vi "Server_API_Call.vi"(6 "Server":path, 7 "Direction":enum16{"ASK", "TELL"}(ring), 8 "error in (no error)":errorcluster, 9 "Payload":string, 11 "cmd":string) -> (0 "error out":errorcluster, 1 "Running?":bool, 3 "Read from Server":string)   [LabVIEW 2020]
panel:
  in  "port":refnum<visa-resource-name>
  out "Script Running?":bool
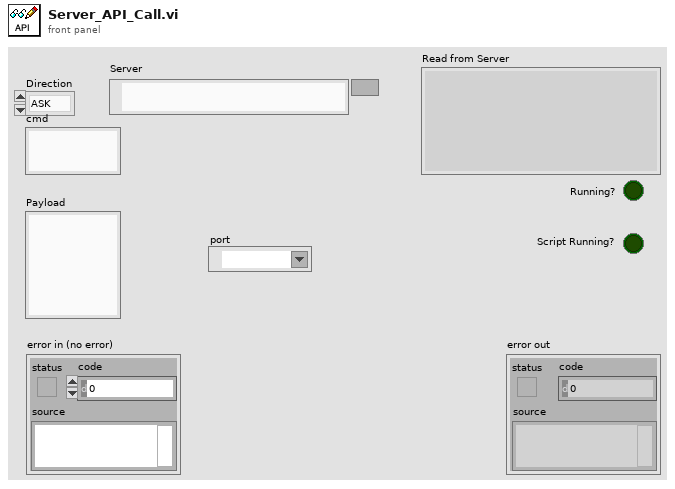
[diagram p1: front panel]
types:
  T1 = enum32{"Bad", "Idle", "Run top level", "Running"}
  T2 = enum32{"Invalid", "Standard", "Closed", "Hidden", "Minimized", "Maximized"}
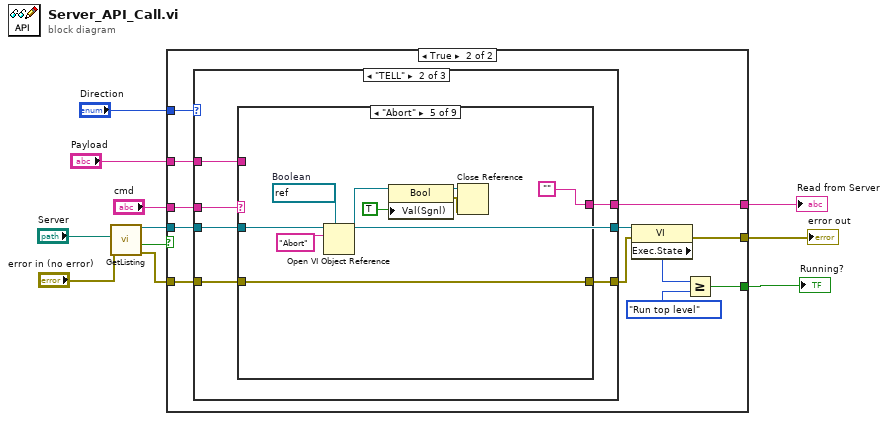
[diagram p0: block diagram]
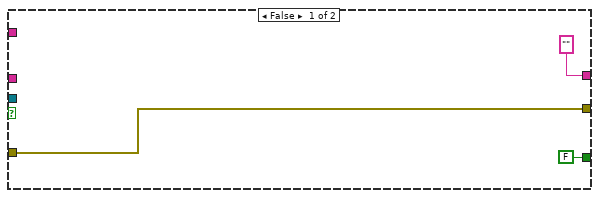
[diagram p2: hidden frame]
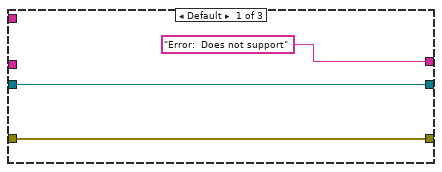
[diagram p3: hidden frame]
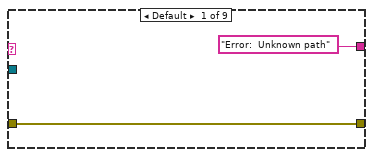
[diagram p4: hidden frame]
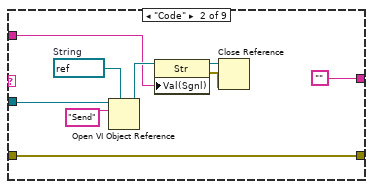
[diagram p5: hidden frame]
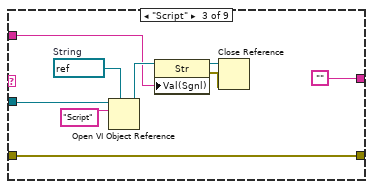
[diagram p6: hidden frame]
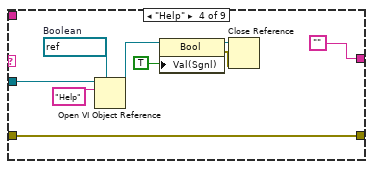
[diagram p7: hidden frame]
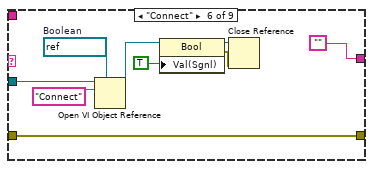
[diagram p8: hidden frame]
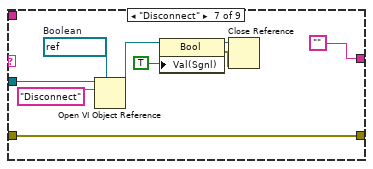
[diagram p9: hidden frame]
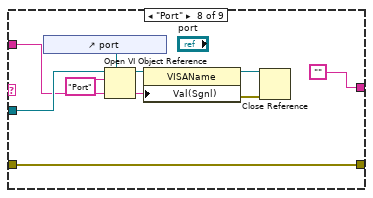
[diagram p10: hidden frame]
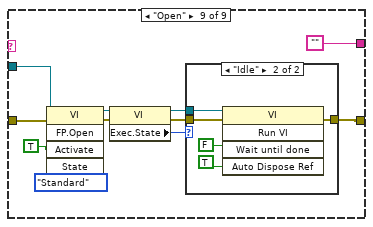
[diagram p11: hidden frame]
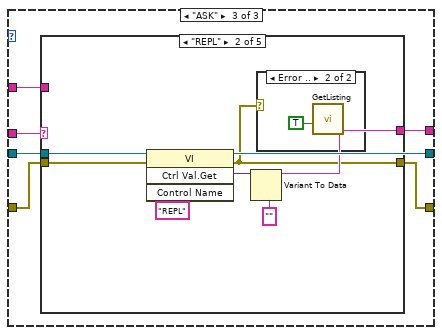
[diagram p13: hidden frame]
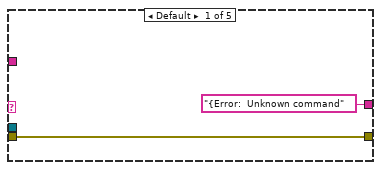
[diagram p14: hidden frame]
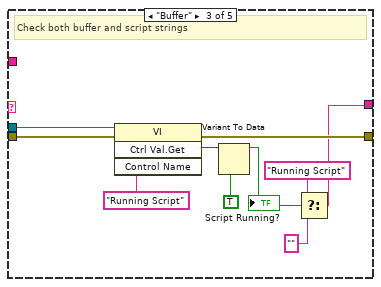
[diagram p16: hidden frame]
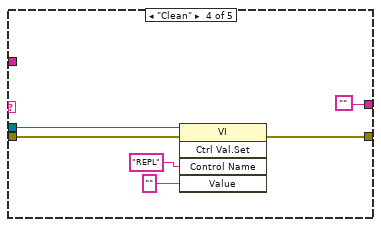
[diagram p17: hidden frame]
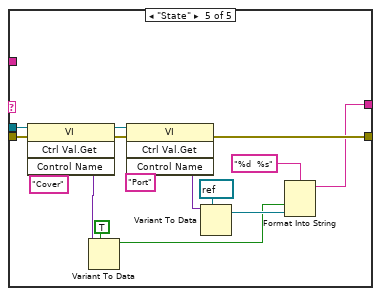
[diagram p18: hidden frame]
diagram:
  n1 = call "GetListing.vi"("error in (no error)"="error in (no error)", "Server"="Server") -> ("error out"=w4:errorcluster, "Found"=w1:bool, "VI out"=w9:refnum<vi>)  [unwired: 7 in]
  n2 = case shown="True" w1 {
    tunnel: ["" ("input 2") w26] -> w11
    tunnel: w9 -> [_ w25]
    tunnel: "Direction" -> [_ w24]
    tunnel: "Payload" -> [_ w23]
    tunnel: "cmd" -> [_ w22]
    tunnel: w4 -> [w13 w21]
    tunnel: [FALSE w16] -> w3
    tunnel: [w13 w15] -> w2
    frame False {
    }
    frame True {
      n3 = case shown="\"TELL\"" w24 {
        tunnel: ["Error:  Does not support" ("input 2") w35 w123] -> w26
        tunnel: w23 -> [_ w34 w122]
        tunnel: w25 -> [w27 w30 w118]
        tunnel: w21 -> [w28 w33 w121]
        tunnel: [w28 w32 w120] -> w19
        tunnel: w22 -> [_ w31 w119]
        tunnel: [w27 w30 w118] -> w20
        frame Default {
        }
        frame "TELL" {
          n4 = case shown="\"Abort\"" w31 {
            tunnel: ["Error:  Unknown path" ("input 2") "" "" "" "" "" "" "" ""] -> w35
            tunnel: w34 -> [_ w40 w49 _ _ _ _ w92 _]
            tunnel: w33 -> [w36 w45 w54 w64 w73 w82 w91 w100 w107]
            tunnel: [w36 w45 w54 w64 w73 w82 w91 w100 w101] -> w32
            tunnel: w30 -> [_ w42 w51 w61 w70 w79 w88 w98 w108]
            frame Default {
            }
            frame "Code" {
              w44 = refnum<vi> refnum  # String
              n5 = Open VI Object Reference(7:w44, 10:"Send" ("name/order"), 11:w42) -> (3:w41:refnum<vi>)  [unwired: 1 in, 1 out]
              n6 = property class="Str"(reference=w41, "Val(Sgnl)"=w40) -> (reference out=w38:refnum<vi>, error out=w39:errorcluster)  [unwired: 1 in]
              n7 = Close Reference(reference=w38, error in (no error)=w39) -> ()  [unwired: 1 out]
            }
            frame "Script" {
              w53 = refnum<vi> refnum  # String
              n8 = Open VI Object Reference(7:w53, 10:"Script" ("name/order"), 11:w51) -> (3:w50:refnum<vi>)  [unwired: 1 in, 1 out]
              n9 = property class="Str"(reference=w50, "Val(Sgnl)"=w49) -> (reference out=w47:refnum<vi>, error out=w48:errorcluster)  [unwired: 1 in]
              n10 = Close Reference(reference=w47, error in (no error)=w48) -> ()  [unwired: 1 out]
            }
            frame "Help" {
              w63 = refnum<vi> refnum  # Boolean
              n11 = Open VI Object Reference(7:w63, 10:"Help" ("name/order"), 11:w61) -> (3:w60:refnum<vi>)  [unwired: 1 in, 1 out]
              n12 = property class="Bool"(reference=w60, "Val(Sgnl)"=TRUE) -> (reference out=w58:refnum<vi>, error out=w59:errorcluster)  [unwired: 1 in]
              n13 = Close Reference(reference=w58, error in (no error)=w59) -> ()  [unwired: 1 out]
            }
            frame "Abort" {
              w72 = refnum<vi> refnum  # Boolean
              n14 = Open VI Object Reference(7:w72, 10:"Abort" ("name/order"), 11:w70) -> (3:w69:refnum<vi>)  [unwired: 1 in, 1 out]
              n15 = property class="Bool"(reference=w69, "Val(Sgnl)"=TRUE) -> (reference out=w67:refnum<vi>, error out=w68:errorcluster)  [unwired: 1 in]
              n16 = Close Reference(reference=w67, error in (no error)=w68) -> ()  [unwired: 1 out]
            }
            frame "Connect" {
              w81 = refnum<vi> refnum  # Boolean
              n17 = Open VI Object Reference(7:w81, 10:"Connect" ("name/order"), 11:w79) -> (3:w78:refnum<vi>)  [unwired: 1 in, 1 out]
              n18 = property class="Bool"(reference=w78, "Val(Sgnl)"=TRUE) -> (reference out=w76:refnum<vi>, error out=w77:errorcluster)  [unwired: 1 in]
              n19 = Close Reference(reference=w76, error in (no error)=w77) -> ()  [unwired: 1 out]
            }
            frame "Disconnect" {
              w90 = refnum<vi> refnum  # Boolean
              n20 = Open VI Object Reference(7:w90, 10:"Disconnect" ("name/order"), 11:w88) -> (3:w87:refnum<vi>)  [unwired: 1 in, 1 out]
              n21 = property class="Bool"(reference=w87, "Val(Sgnl)"=TRUE) -> (reference out=w85:refnum<vi>, error out=w86:errorcluster)  [unwired: 1 in]
              n22 = Close Reference(reference=w85, error in (no error)=w86) -> ()  [unwired: 1 out]
            }
            frame "Port" {
              n23 = control-ref of="port"() -> (w93:refnum<vi>)
              n24 = Open VI Object Reference(7:w93, 10:"Port" ("name/order"), 11:w98) -> (3:w97:refnum<vi>)  [unwired: 1 in, 1 out]
              n25 = property class="VISAName"(reference=w97, "Val(Sgnl)"=w92) -> (reference out=w95:refnum<vi>, error out=w96:errorcluster)  [unwired: 1 in]
              n26 = Close Reference(reference=w95, error in (no error)=w96) -> ()  [unwired: 1 out]
            }
            frame "Open" {
              n27 = invoke class="VI" method="FP.Open"(reference=w108, error in=w107, "Activate"=TRUE ("Activate?"), "State"=T2."Standard" ("Front Panel Window:State")) -> (reference out=w106:refnum<vi>, error out=w105:errorcluster)  [unwired: 1 in, 3 out]
              n28 = property class="VI"(reference=w106, error in=w105) -> (reference out=w103:refnum<vi>, error out=w102:errorcluster, "Exec.State"=w104:T1)
              n29 = case shown="\"Idle\"" w104 {
                tunnel: w103 -> [_ w117]
                tunnel: w102 -> [w112 w116]
                tunnel: [w112 w115] -> w101
                frame Default {
                }
                frame "Idle" {
                  n30 = invoke class="VI" method="Run VI"(reference=w117, error in=w116, "Wait until done"=FALSE ("Activate?"), "Auto Dispose Ref"=TRUE ("Activate?")) -> (error out=w115:errorcluster)  [unwired: 1 in, 4 out]
                }
              }
            }
          }
        }
        frame "ASK" {
          n31 = case shown="\"REPL\"" w119 {
            tunnel: ["{Error:  Unknown command" ("input 2") w127 w135 "" w150] -> w123
            tunnel: w122 -> [_ _ _ _ _]
            tunnel: w118 -> [_ w128 w140 w146 w158]
            tunnel: w121 -> [w124 w129 w134 w145 w157]
            tunnel: [w124 w126 w141 w144 w154] -> w120
            frame Default {
            }
            frame "REPL" {
              n32 = invoke class="VI" method="Ctrl Val.Get"(reference=w128, error in=w129, "Control Name"="REPL") -> (error out=w126:errorcluster, "Get Control Value Variant"=w131:variant)  [unwired: 1 in, 2 out]
              n33 = Variant To Data(type="" ("Control Name"), Variant=w131) -> (data=w127:string)  [unwired: 1 in, 1 out]
              n34 = case shown="Error .." w126 {
                frame No Error {
                }
                frame Error {
                  n35 = call "GetListing.vi"("Reset?"=TRUE) -> ()  [unwired: 8 in, 3 out]
                }
              }
            }
            frame "Buffer" {
              # "Check both buffer and script strings"
              n36 = invoke class="VI" method="Ctrl Val.Get"(reference=w140, error in=w134, "Control Name"="Running Script") -> (error out=w141:errorcluster, "Get Control Value Variant"=w142:variant)  [unwired: 1 in, 2 out]
              n37 = Variant To Data(type=TRUE, Variant=w142) -> (data=w138:bool)  [unwired: 1 in, 1 out]
              "Script Running?" <- w138
              n38 = Select(t="Running Script" ("Control Name"), s=w138, f="" ("Control Name")) -> (s? t:f=w135:string)
            }
            frame "Clean" {
              n39 = invoke class="VI" method="Ctrl Val.Set"(reference=w146, error in=w145, "Control Name"="REPL", "Value"="" ("Control Name")) -> (error out=w144:errorcluster)  [unwired: 1 in, 4 out]
            }
            frame "State" {
              n40 = invoke class="VI" method="Ctrl Val.Get"(reference=w158, error in=w157, "Control Name"="Cover") -> (reference out=w156:refnum<vi>, error out=w155:errorcluster, "Get Control Value Variant"=w159:variant)  [unwired: 1 in, 1 out]
              n41 = Variant To Data(type=TRUE, Variant=w159) -> (data=w151:bool)  [unwired: 1 in, 1 out]
              n42 = invoke class="VI" method="Ctrl Val.Get"(reference=w156, error in=w155, "Control Name"="Port") -> (error out=w154:errorcluster, "Get Control Value Variant"=w160:variant)  [unwired: 1 in, 2 out]
              n43 = Variant To Data(type=refnum<visa-resource-name> refnum ("Port"), Variant=w160) -> (data=w153:refnum<visa-resource-name>)  [unwired: 1 in, 1 out]
              n44 = Format Into String(format string="%d  %s", w151, w153) -> (resulting string=w150:string)  [unwired: 2 in, 1 out]
            }
          }
        }
      }
      n45 = property class="VI"(reference=w20, error in=w19) -> (error out=w15:errorcluster, "Exec.State"=w18:T1)  [unwired: 1 out]
      n46 = Greater Or Equal?(x=w18, y=T1."Run top level" ("Execution:State")) -> (x >= y?=w16:bool)
    }
  }
  "error out" <- w2
  "Read from Server" <- w11
  "Running?" <- w3
